vi "Test Parse ISO 8601 Timestamps.vi"(8 "error in (no error)":errorcluster) -> (0 "error out":errorcluster)   [LabVIEW 2020]
uses:
  <vilib>/addons/_JKI Toolkits/Caraya/classes/Test/Test.lvclass
  <vilib>/addons/_JKI Toolkits/Caraya/classes/Assert/Assert.lvclass
  src/Deserializer/JSON Deserializer/JSON Deserializer.lvclass
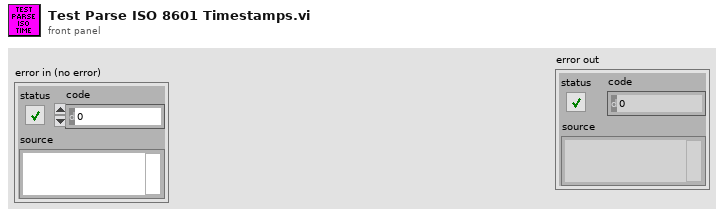
[diagram p1: front panel]
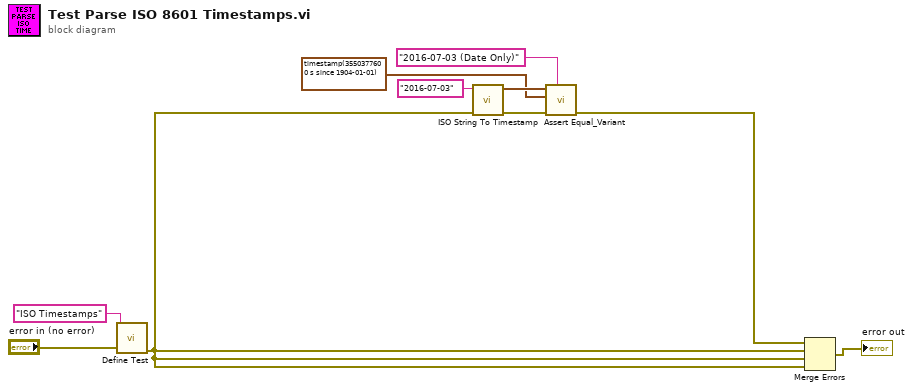
[diagram p0: block diagram]
diagram:
  n1 = call <vilib>:"Define Test.vi"("error in (no error)"="error in (no error)", "Label (VI Title)"="ISO Timestamps") -> ("error out"=w1:errorcluster)  [unwired: 8 in, 1 out]
  n2 = call "ISO String To Timestamp.vi"("error in (no error)"=w1, "ISO Timestamp String"="2016-07-03") -> ("error out"=w4:errorcluster, "Time Stamp"=w3:timestamp)  [unwired: 8 in]
  n3 = call <vilib>:"Assert Equal_Variant.vi"("Label"="2016-07-03 (Date Only)", "error in (no error)"=w4, "Y"=timestamp(3550377600 s since 1904-01-01) ("Time Stamp"), "X"=w3) -> ("error out"=w7:errorcluster)  [unwired: 7 in]
  n4 = Merge Errors(w7, w1, w1, w1) -> (→"error out":errorcluster)
